vi "HSL to RGB.vi"(8 "error in (no error)":errorcluster, 9 "Lightness(%)":dbl format="%#_13g", 10 "Saturation(%)":dbl format="%#_13g", 11 "Hue(°)":dbl format="%#_13g") -> (0 "error out":errorcluster, 1 "Blue":u8, 2 "Green":u8, 3 "Red":u8)   [LabVIEW 2018, in "Colour Lab.lvlib"]
uses:
  Colour Lab.lvlib
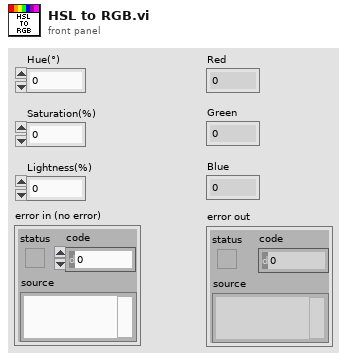
[diagram p1: front panel]
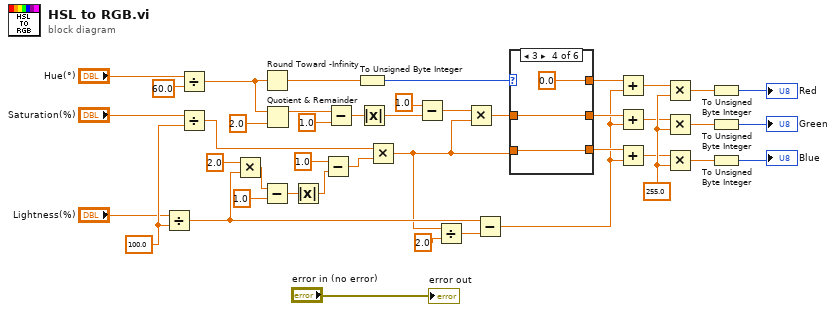
[diagram p0: block diagram]
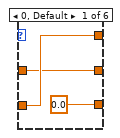
[diagram p2: hidden frame]
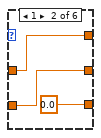
[diagram p3: hidden frame]
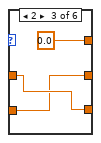
[diagram p4: hidden frame]
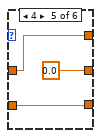
[diagram p5: hidden frame]
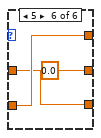
[diagram p6: hidden frame]
diagram:
  w18 = 100.0 ("y")
  w27 = 255.0 ("y")
  n1 = Divide(x="Lightness(%)", y=w18) -> (x/y=w11:dbl)
  n2 = Divide(x="Hue(°)", y=60.0) -> (x/y=w33:dbl)
  n3 = Divide(x="Saturation(%)", y=w18) -> (x/y=w19:dbl)
  n4 = Multiply(x=2.0 ("y"), y=w11) -> (x*y=w12:dbl)
  n5 = Round Toward -Infinity(1:w33) -> (0:w32:dbl)
  n6 = Subtract(x=w12, y=1.0) -> (x-y=w14:dbl)
  n7 = Quotient & Remainder(x=w33, y=2.0) -> (x-y*floor(x/y)=w36:dbl)  [unwired: 1 out]
  n8 = Absolute Value(x=w14) -> (abs(x)=w15:dbl)
  n9 = Subtract(x=1.0, y=w15) -> (x-y=w17:dbl)
  n10 = Subtract(x=w36, y=1.0) -> (x-y=w38:dbl)
  n11 = To Unsigned Byte Integer(number=w32) -> (unsigned 8bit integer=w31:u8)
  n12 = Absolute Value(x=w38) -> (abs(x)=w39:dbl)
  n13 = Multiply(x=w19, y=w17) -> (x*y=w9:dbl)
  n14 = Subtract(x=1.0, y=w39) -> (x-y=w41:dbl)
  n15 = Divide(x=w9, y=2.0) -> (x/y=w8:dbl)
  n16 = Multiply(x=w41, y=w9) -> (x*y=w34:dbl)
  n17 = Subtract(x=w11, y=w8) -> (x-y=w22:dbl)
  n18 = case shown="3" w31 {
    tunnel: w9 -> [w46 w48 w50 w54 w57 w61]
    tunnel: w34 -> [w45 w49 w51 w55 w58 w59]
    tunnel: [0.0 0.0 w51 w54 w57 w59] -> w23
    tunnel: [w45 w48 w50 w55 0.0 0.0] -> w24
    tunnel: [w46 w49 0.0 0.0 w58 w61] -> w25
    frame 0, Default {
    }
    frame 1 {
    }
    frame 2 {
    }
    frame 3 {
    }
    frame 4 {
    }
    frame 5 {
    }
  }
  n19 = Add(x=w25, y=w22) -> (x+y=w26:dbl)
  n20 = Add(x=w24, y=w22) -> (x+y=w20:dbl)
  n21 = Add(x=w23, y=w22) -> (x+y=w21:dbl)
  n22 = Multiply(x=w26, y=w27) -> (x*y=w30:dbl)
  n23 = Multiply(x=w20, y=w27) -> (x*y=w29:dbl)
  n24 = Multiply(x=w21, y=w27) -> (x*y=w28:dbl)
  n25 = To Unsigned Byte Integer(number=w30) -> (unsigned 8bit integer=→"Red":u8)
  n26 = To Unsigned Byte Integer(number=w29) -> (unsigned 8bit integer=→"Green":u8)
  n27 = To Unsigned Byte Integer(number=w28) -> (unsigned 8bit integer=→"Blue":u8)
  "error out" <- "error in (no error)"
